vi "5T_Merge_Cluster.vi"(1 "5T Control":T2 {"Rate (T/min)" format="%6_5f"}, 2 "5 T Status":T3 {"Leads (T)" format="%#_6f"}) -> (0 "5 T Cluster":T1 {"Rate (T/min)" format="%6_5f"; "Leads (T)" format="%6_5f"})   [LabVIEW 2019]
uses:
  Mischer/5T_Status.ctl
  Mischer/5T_Control.ctl
  Mischer/5T-Cluster.ctl
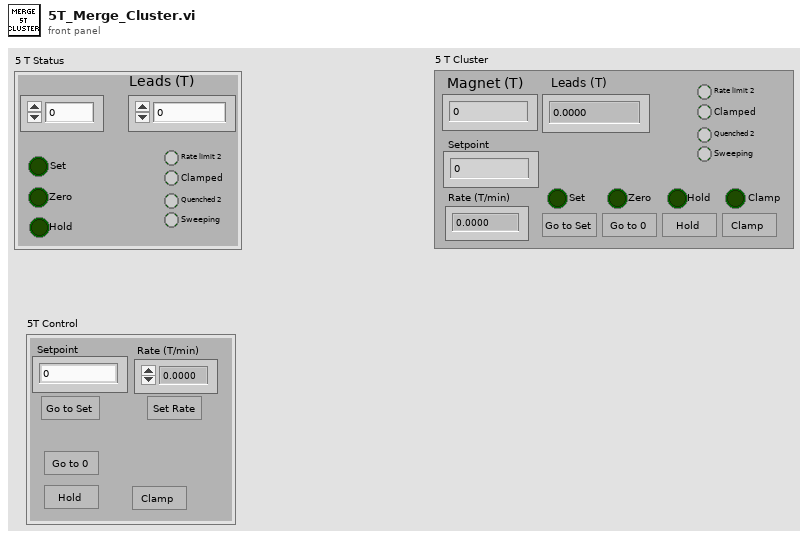
[diagram p1: front panel]
types:
  T1 = typedef "5T-Cluster.ctl" = cluster{"Go to set":bool, "Go to Zero":bool, "Clamp":bool, "Go to Hold":bool, "Clamped ":bool, "Quenched 2":bool, "Rate limit 2":bool, "Magnet (T)":dbl, "Leads (T)":dbl, "Rate (T/min)":dbl, "Sweeping":bool, "Setpoint":dbl, "Set":bool, "Zero":bool, "Hold":bool, "Clamp":bool}
  T2 = typedef "5T_Control.ctl" = cluster{"Rate (T/min)":dbl, "Setpoint":dbl, "Go to set":bool, "Go to Zero":bool, "Clamp":bool, "Go to Hold":bool, "Set Rate":bool}
  T3 = typedef "5T_Status.ctl" = cluster{"Magnet (T)":dbl, "Leads (T)":dbl, "Clamped ":bool, "Quenched 2":bool, "Rate limit 2":bool, "Sweeping":bool, "Set":bool, "Zero":bool, "Hold":bool}
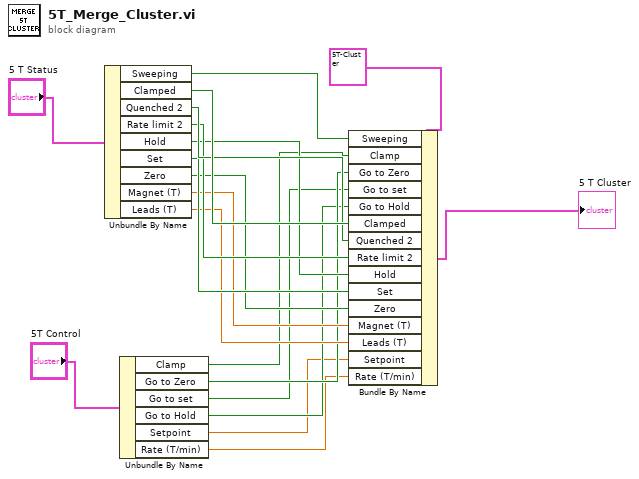
[diagram p0: block diagram]
diagram:
  n1 = Unbundle By Name("5 T Status") -> ("Sweeping"=w15:bool, "Clamped"=w14:bool, "Quenched 2"=w13:bool, "Rate limit 2"=w12:bool, "Hold"=w11:bool, "Set"=w10:bool, "Zero"=w9:bool, "Magnet (T)"=w8:dbl, "Leads (T)"=w7:dbl)
  n2 = Unbundle By Name("5T Control") -> ("Clamp"=w6:bool, "Go to Zero"=w5:bool, "Go to set"=w4:bool, "Go to Hold"=w3:bool, "Setpoint"=w2:dbl, "Rate (T/min)"=w1:dbl)
  n3 = Bundle By Name(cluster=T1 {"Go to set"=FALSE, "Go to Zero"=FALSE, "Clamp"=FALSE, "Go to Hold"=FALSE, "Clamped "=FALSE, "Quenched 2"=FALSE, "Rate limit 2"=FALSE, "Magnet (T)"=0.0, "Leads (T)"=0.0, "Rate (T/min)"=0.0, "Sweeping"=FALSE, "Setpoint"=0.0, "Set"=FALSE, "Zero"=FALSE, "Hold"=FALSE, "Clamp"=FALSE} ("5 T Cluster"), "Sweeping"=w15, "Clamp"=w6, "Go to Zero"=w5, "Go to set"=w4, "Go to Hold"=w3, "Clamped"=w14, "Quenched 2"=w13, "Rate limit 2"=w12, "Hold"=w11, "Set"=w10, "Zero"=w9, "Magnet (T)"=w8, "Leads (T)"=w7, "Setpoint"=w2, "Rate (T/min)"=w1) -> (→"5 T Cluster":T1)
